vi "lpString to lvString.vi"(11 "LPTSTR String":string) -> (3 "LVString":string)   [LabVIEW 2017, in "BonTechDetector.lvlib"]
uses:
  BonTechDetector.lvlib
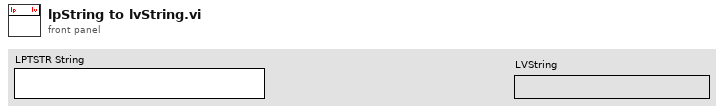
[diagram p1: front panel]
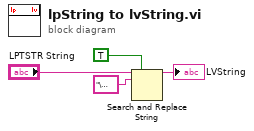
[diagram p0: block diagram]
diagram:
  n1 = Search and Replace String(replace all?=TRUE ("replace all? (F)"), input string="LPTSTR String", search string="\u0000") -> (result string=→"LVString":string)  [unwired: 5 in, 3 out]
